vi "ReleaseSensorInstance.vi"(0 "Fehler (Eingang, kein Fehler)":errorcluster, 5 "instanceHandle":u32, 7 "DLL-Path":path) -> (4 "Fehler (Ausgang)":errorcluster, 6 "instanceHandle":u32, 8 "DLL-Path":path, 10 "ERR_CODE":i32)   [LabVIEW 2015, in "MEDAQLib.lvlib"]
doc: "ERR_CODE ReleaseSensorInstance (DWORD instanceHandle);\n\nClose the driver, free all sensor instances."
uses:
  MEDAQLib.lvlib
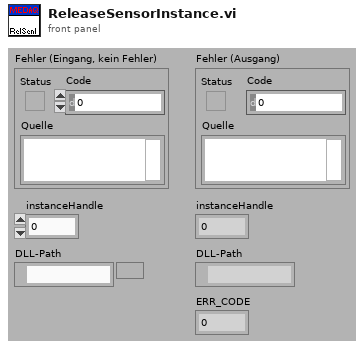
[diagram p1: front panel]
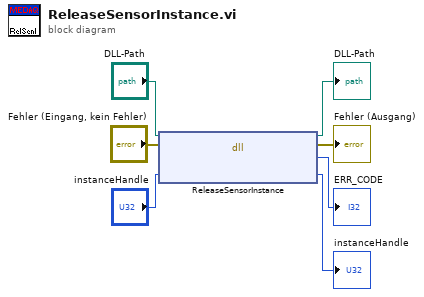
[diagram p0: block diagram]
diagram:
  n1 = dll-call lib="D:/Users/XRF/Desktop/Dante_acquire6/libs/Proximity_sensor/Release/MEDAQLib.dll" fn="ReleaseSensorInstance"(path in="DLL-Path", error in="Fehler (Eingang, kein Fehler)", "instanceHandle"="instanceHandle") -> (path out=→"DLL-Path":path, error out=→"Fehler (Ausgang)":errorcluster, "Rückgabetyp"=→"ERR_CODE":i32, "instanceHandle"=→"instanceHandle":u32)  [unwired: 1 in]
